vi "widget.vi"(7 "LabVIEW Web Service Request":refnum<class "Web Request.lvclass">, 10 "widget_name":string, 11 "context_id":string) -> (3 "url":string)   [LabVIEW 2013]
uses:
  <vilib>/wsapi/Web Request.lvclass
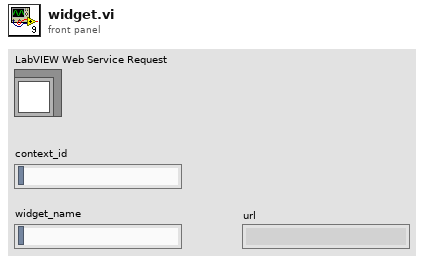
[diagram p1: front panel]
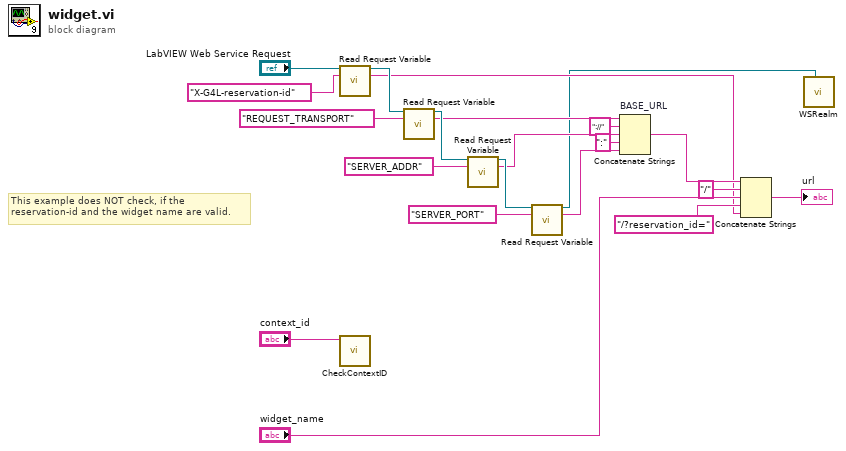
[diagram p0: block diagram]
diagram:
  # "This example does NOT check, if the\nreservation-id and the widget name are valid."
  n1 = call <vilib>:"Read Request Variable.vi"("LabVIEW Web Service Request"="LabVIEW Web Service Request", "variable name"="X-G4L-reservation-id") -> ("LabVIEW Web Service Request out"=w13:refnum<class "Web Request.lvclass">, "value"=w3:string)  [unwired: 11 in, 1 out]
  n2 = call "CheckContextID.vi"("context_id"="context_id") -> ()  [unwired: 10 in, 1 out]
  n3 = call <vilib>:"Read Request Variable.vi"("LabVIEW Web Service Request"=w13, "variable name"="REQUEST_TRANSPORT") -> ("LabVIEW Web Service Request out"=w15:refnum<class "Web Request.lvclass">, "value"=w12:string)  [unwired: 11 in, 1 out]
  n4 = call <vilib>:"Read Request Variable.vi"("LabVIEW Web Service Request"=w15, "variable name"="SERVER_ADDR") -> ("LabVIEW Web Service Request out"=w14:refnum<class "Web Request.lvclass">, "value"=w10:string)  [unwired: 11 in, 1 out]
  n5 = call <vilib>:"Read Request Variable.vi"("LabVIEW Web Service Request"=w14, "variable name"="SERVER_PORT") -> ("LabVIEW Web Service Request out"=w2:refnum<class "Web Request.lvclass">, "value"=w8:string)  [unwired: 11 in, 1 out]
  n6 = Concatenate Strings "BASE_URL"(w12, "://" ("string"), w10, ":" ("string"), w8) -> (w7:string)
  n7 = Concatenate Strings(w7, "/" ("string"), "widget_name", "/?reservation_id=" ("string"), w3) -> (→"url":string)
  n8 = call "WSRealm.vi"("LabVIEW Web Service Request"=w2) -> ()  [unwired: 11 in]
